vi "formatExtentData.vi"(11 "extent":T1[](array[typedef])=[{"X"=0.0, "Y"=0.0, "Z"=0.0}, {"X"=0.0, "Y"=0.0, "Z"=0.0}]) -> (3 "formatedExtentData":string)   [LabVIEW 2015]
uses:
  <vilib>/Utility/miscctls.llb/LV3DPointTypeDef.ctl
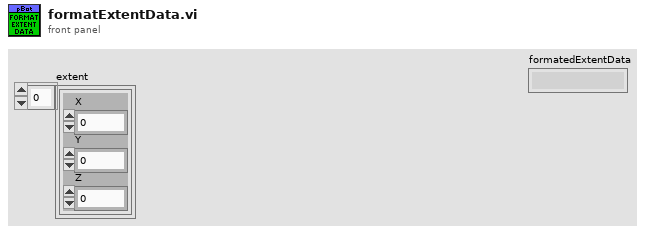
[diagram p1: front panel]
types:
  T1 = typedef "LV3DPointTypeDef.ctl" = cluster{"X":sgl, "Y":sgl, "Z":sgl}
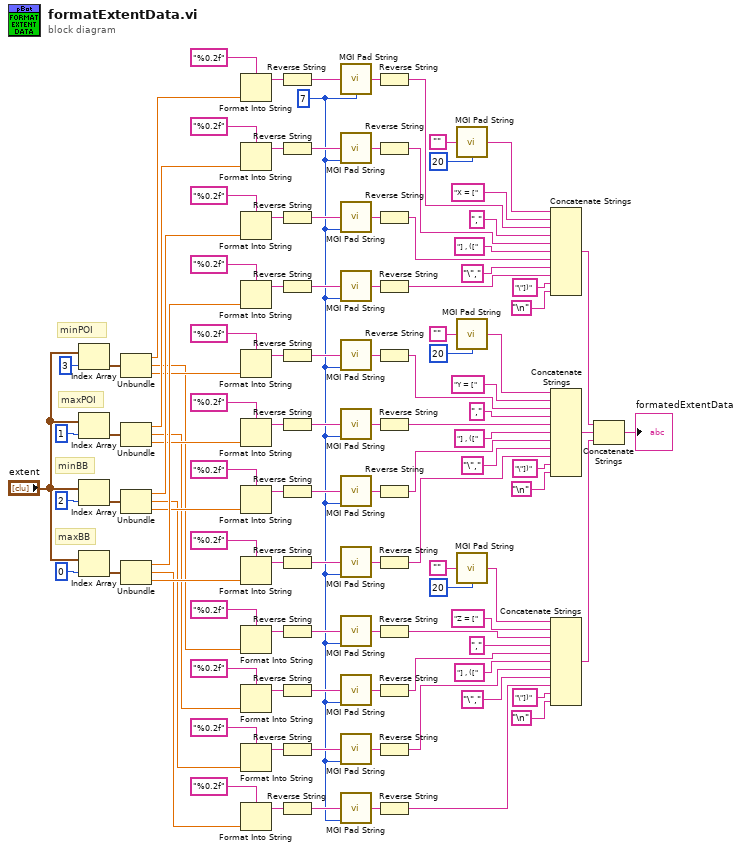
[diagram p0: block diagram]
diagram:
  w1 = u32 7 ("End Length")
  # "minBB"
  # "maxBB"
  # "minPOI"
  # "maxPOI"
  n1 = Index Array(array="extent", index=3) -> (element=w112:T1)
  n2 = Index Array(array="extent", index=1) -> (element=w113:T1)
  n3 = Index Array(array="extent", index=2) -> (element=w108:T1)
  n4 = Index Array(array="extent", index=0) -> (element=w107:T1)
  n5 = Unbundle(w112) -> ("X"=w17:sgl, "Y"=w6:sgl, "Z"=w10:sgl)
  n6 = Unbundle(w113) -> ("X"=w16:sgl, "Y"=w7:sgl, "Z"=w11:sgl)
  n7 = Unbundle(w108) -> ("X"=w15:sgl, "Y"=w8:sgl, "Z"=w12:sgl)
  n8 = Unbundle(w107) -> ("X"=w14:sgl, "Y"=w9:sgl, "Z"=w13:sgl)
  n9 = Format Into String(format string="%0.2f", w17) -> (resulting string=w98:string)  [unwired: 2 in, 1 out]
  n10 = Format Into String(format string="%0.2f", w16) -> (resulting string=w97:string)  [unwired: 2 in, 1 out]
  n11 = Format Into String(format string="%0.2f", w15) -> (resulting string=w91:string)  [unwired: 2 in, 1 out]
  n12 = Format Into String(format string="%0.2f", w14) -> (resulting string=w90:string)  [unwired: 2 in, 1 out]
  n13 = Format Into String(format string="%0.2f", w10) -> (resulting string=w53:string)  [unwired: 2 in, 1 out]
  n14 = Format Into String(format string="%0.2f", w11) -> (resulting string=w54:string)  [unwired: 2 in, 1 out]
  n15 = Format Into String(format string="%0.2f", w12) -> (resulting string=w60:string)  [unwired: 2 in, 1 out]
  n16 = Format Into String(format string="%0.2f", w13) -> (resulting string=w61:string)  [unwired: 2 in, 1 out]
  n17 = Format Into String(format string="%0.2f", w6) -> (resulting string=w40:string)  [unwired: 2 in, 1 out]
  n18 = Format Into String(format string="%0.2f", w7) -> (resulting string=w39:string)  [unwired: 2 in, 1 out]
  n19 = Format Into String(format string="%0.2f", w8) -> (resulting string=w33:string)  [unwired: 2 in, 1 out]
  n20 = Format Into String(format string="%0.2f", w9) -> (resulting string=w32:string)  [unwired: 2 in, 1 out]
  n21 = Reverse String(1:w98) -> (0:w100:string)
  n22 = Reverse String(1:w97) -> (0:w95:string)
  n23 = Reverse String(1:w91) -> (0:w93:string)
  n24 = Reverse String(1:w90) -> (0:w88:string)
  n25 = Reverse String(1:w53) -> (0:w51:string)
  n26 = Reverse String(1:w54) -> (0:w56:string)
  n27 = Reverse String(1:w60) -> (0:w58:string)
  n28 = Reverse String(1:w61) -> (0:w63:string)
  n29 = Reverse String(1:w40) -> (0:w42:string)
  n30 = Reverse String(1:w39) -> (0:w37:string)
  n31 = Reverse String(1:w33) -> (0:w35:string)
  n32 = Reverse String(1:w32) -> (0:w30:string)
  n33 = call <userlib>:"MGI Pad String.vi"("String In"=w100, "End Length"=w1) -> ("String Out"=w99:string)  [unwired: 13 in]
  n34 = call <userlib>:"MGI Pad String.vi"("String In"=w95, "End Length"=w1) -> ("String Out"=w96:string)  [unwired: 13 in]
  n35 = call <userlib>:"MGI Pad String.vi"("String In"=w93, "End Length"=w1) -> ("String Out"=w92:string)  [unwired: 13 in]
  n36 = call <userlib>:"MGI Pad String.vi"("String In"=w88, "End Length"=w1) -> ("String Out"=w89:string)  [unwired: 13 in]
  n37 = call <userlib>:"MGI Pad String.vi"("String In"=w51, "End Length"=w1) -> ("String Out"=w52:string)  [unwired: 13 in]
  n38 = call <userlib>:"MGI Pad String.vi"("String In"=w56, "End Length"=w1) -> ("String Out"=w55:string)  [unwired: 13 in]
  n39 = call <userlib>:"MGI Pad String.vi"("String In"=w58, "End Length"=w1) -> ("String Out"=w59:string)  [unwired: 13 in]
  n40 = call <userlib>:"MGI Pad String.vi"("String In"=w63, "End Length"=w1) -> ("String Out"=w62:string)  [unwired: 13 in]
  n41 = call <userlib>:"MGI Pad String.vi"("String In"=w42, "End Length"=w1) -> ("String Out"=w41:string)  [unwired: 13 in]
  n42 = call <userlib>:"MGI Pad String.vi"("String In"=w37, "End Length"=w1) -> ("String Out"=w38:string)  [unwired: 13 in]
  n43 = call <userlib>:"MGI Pad String.vi"("String In"=w35, "End Length"=w1) -> ("String Out"=w34:string)  [unwired: 13 in]
  n44 = call <userlib>:"MGI Pad String.vi"("String In"=w30, "End Length"=w1) -> ("String Out"=w31:string)  [unwired: 13 in]
  n45 = Reverse String(1:w99) -> (0:w84:string)
  n46 = Reverse String(1:w96) -> (0:w82:string)
  n47 = Reverse String(1:w92) -> (0:w80:string)
  n48 = Reverse String(1:w89) -> (0:w78:string)
  n49 = Reverse String(1:w52) -> (0:w67:string)
  n50 = Reverse String(1:w55) -> (0:w69:string)
  n51 = Reverse String(1:w59) -> (0:w71:string)
  n52 = Reverse String(1:w62) -> (0:w73:string)
  n53 = Reverse String(1:w41) -> (0:w26:string)
  n54 = Reverse String(1:w38) -> (0:w24:string)
  n55 = Reverse String(1:w34) -> (0:w22:string)
  n56 = Reverse String(1:w31) -> (0:w20:string)
  n57 = call <userlib>:"MGI Pad String.vi"("String In"="", "End Length"=u32 20) -> ("String Out"=w101:string)  [unwired: 13 in]
  n58 = call <userlib>:"MGI Pad String.vi"("String In"="", "End Length"=u32 20) -> ("String Out"=w50:string)  [unwired: 13 in]
  n59 = call <userlib>:"MGI Pad String.vi"("String In"="", "End Length"=u32 20) -> ("String Out"=w43:string)  [unwired: 13 in]
  n60 = Concatenate Strings(w101, "X = [" ("format string"), w84, "," ("format string"), w82, "] , ([" ("format string"), w80, "\"," ("string"), w78, "\"])" ("string"), "\n") -> (w4:string)
  n61 = Concatenate Strings(w50, "Y = [" ("format string"), w67, "," ("format string"), w69, "] , ([" ("format string"), w71, "\"," ("string"), w73, "\"])" ("string"), "\n") -> (w5:string)
  n62 = Concatenate Strings(w43, "Z = [" ("format string"), w26, "," ("format string"), w24, "] , ([" ("format string"), w22, "\"," ("string"), w20, "\"])" ("string"), "\n") -> (w3:string)
  n63 = Concatenate Strings(w4, w5, w3) -> (→"formatedExtentData":string)
